vi "Gasteiler_Standby.vi"   [LabVIEW 2020, in "Linearisierung v2.lvlib"]
uses:
  Linearisierung v2.lvlib
  Gasteiler/Aktionen FGV Gasteiler Daten.ctl
  Gasteiler/AK-Komm Gasteiler/Aktionen AK Komm.ctl
  Gasteiler/Horiba/Aktion Befehl.ctl
  Gasteiler/AK-Komm Gasteiler/Alter Gasteiler/Aktionen AK Komm_ALT.ctl
  Gasteiler/AK-Komm Gasteiler/AK Komm Gasteiler.lvlib
  Gasteiler/Horiba/Horiba GDC.lvlib
  Gasteiler/AK-Komm Gasteiler/Alter Gasteiler/Alter Gasteiler.lvlib
  Gasteiler/Gasteiler.lvlib
types:
  T1 = typedef "Linearisierung v2.lvlib/Gasteiler.lvlib/Aktionen FGV Gasteiler Daten.ctl" = enum16{"lesen", "Gasteiler Daten", "Seriellen Param.", "MB-Endwert", "laden", "speichern", "Anforderung", "TCP", "Aufzeichnung Start"}
  T2 = typedef "Linearisierung v2.lvlib/GasteilerType.ctl" = u16
  T3 = typedef "Linearisierung v2.lvlib/Gasteiler.lvlib/AK Komm Gasteiler.lvlib/Aktionen AK Komm.ctl" = enum16{"lesen", "initialisieren", "beenden", "Status", "SMAN", "SREM", "STBY", "ASTF", "ASTZ", "SLST", "AGAT", "EGAK", "AGAK", "AKAK", "ADRU", "SKOP", "SVSA", "SVSZ", "SONO", "SAIR", "SNOX", "ANOX", "SSPL", "SRUC", "SLIN", "ALST", "ETYP", "SVIO", "LCYL", "CCYL", "DCYL", "SCYL", "GCYL", "DRGV", "DRDC"}
  T4 = typedef "Linearisierung v2.lvlib/Gasteiler.lvlib/Horiba GDC.lvlib/Aktion Befehl.ctl" = enum16{"lesen", "initialisieren", "Beenden", "Standby", "GD/CC", "Info", "Flow", "Alarm", "GD parameter", "GD point", "Durchfluss", "Spuelen1", "Spuelen1 On", "Spuelen1Off", "Spuelen2", "Ventil-Abfrage", "Reset"}
  T5 = typedef "Linearisierung v2.lvlib/Gasteiler.lvlib/AK Komm Gasteiler.lvlib/Alter Gasteiler.lvlib/Aktionen AK Komm_ALT.ctl" = enum16{"lesen", "initialisieren", "beenden", "SRES", "STBY", "SREM", "SMAN", "SLIN", "SLCH", "SLST", "SSPL", "AGAT", "ALST", "ASTZ", "ASTF", "AGAK", "EGAK"}
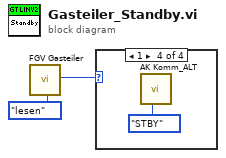
[diagram p0: block diagram]
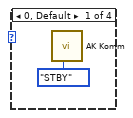
[diagram p2: hidden frame]
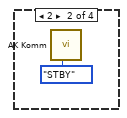
[diagram p3: hidden frame]
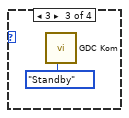
[diagram p4: hidden frame]
diagram:
  n1 = call "FGV Gasteiler.vi"("Aktionen"=Aktionen_FGV_Gasteiler_Daten."lesen") -> ("Gasteiler Type"=w1:T2)  [unwired: 11 in, 7 out]
  n2 = case shown="1" w1 {
    frame 0, Default {
      n3 = call "AK Komm.vi"("Aktionen"=Aktionen_AK_Komm."STBY") -> ()  [unwired: 4 in, 7 out]
    }
    frame 2 {
      n4 = call "AK Komm.vi"("Aktionen"=Aktionen_AK_Komm."STBY") -> ()  [unwired: 4 in, 7 out]
    }
    frame 3 {
      n5 = call "GDC Kom.vi"("Befehl"=Aktion_Befehl."Standby") -> ()  [unwired: 4 in, 7 out]
    }
    frame 1 {
      n6 = call "AK Komm_ALT.vi"("Aktionen_ALT"=Aktionen_AK_Komm_ALT."STBY") -> ()  [unwired: 6 in, 5 out]
    }
  }
